vi "Add Points to Series_DBL.vi"(6 "YValuesPerPoint":i32=1, 8 "error in (no error)":errorcluster, 9 "Data":dbl[](array[numeric]), 10 ".NET MSChart Series":refnum<k24>) -> (0 "error out":errorcluster)   [LabVIEW 2015, in "Graph Extensions MSChart.lvlib"]
uses:
  Graph Extensions MSChart.lvlib
  System.Windows.Forms.DataVisualization
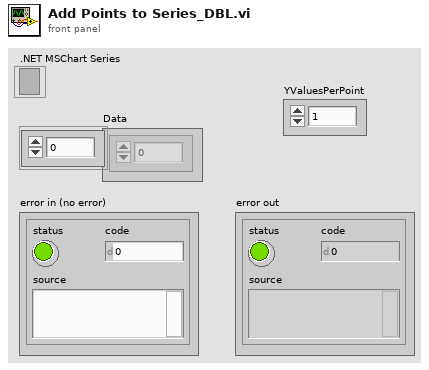
[diagram p1: front panel]
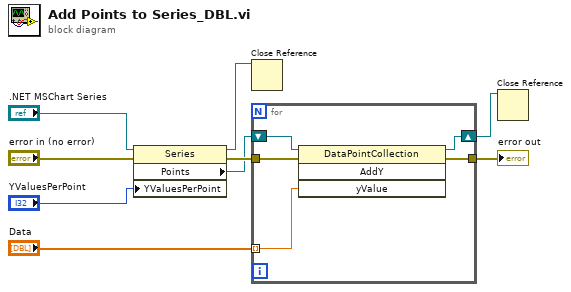
[diagram p0: block diagram]
diagram:
  n1 = property class="Series"(reference=".NET MSChart Series", error in="error in (no error)", "YValuesPerPoint"="YValuesPerPoint") -> (reference out=w2:refnum<k24>, error out=w5:errorcluster, "Points"=w4:refnum<k24>)
  n2 = Close Reference(reference=w2) -> ()  [unwired: 1 in, 1 out]
  n3 = for {
    tunnel: "Data" -> [w13] mode=indexing
    tunnel: [w11] -> w9
    shift-right: [w12] -> w1
    shift-left: w4 -> [w14]
    tunnel: w5 -> [w10]
    n4 = invoke class="DataPointCollection" method="AddY"(reference=w14, error in=w10, "yValue"=w13) -> (reference out=w12:refnum<k24>, error out=w11:errorcluster)  [unwired: 1 in, 2 out]
  }
  "error out" <- w9
  n5 = Close Reference(reference=w1) -> ()  [unwired: 1 in, 1 out]
